vi "RFID Read Example.vi"() -> ()   [LabVIEW 2012, in "Phidget RFID.lvlib"]
uses:
  <instrlib>/Phidgets/Phidget RFID/Phidget RFID.lvlib
  <instrlib>/Phidgets/Phidget RFID/Public/RFIDStart.vi
  <instrlib>/Phidgets/Phidget RFID/Public/RFIDClose.vi
  <instrlib>/Phidgets/Phidget Common/Phidget Common.lvlib
panel:
  out "Protocol":i32(ring) items=["PROTOCOL_EM4100"=1, "PROTOCOL_ISO11785_FDX_B"=2, "PROTOCOL_PHIDGETS"=3]
  out "Tag String":string
  out "Tag Present":bool caption="Tag State"
  in  "stop":bool
  out "error out":errorcluster
  in  "error in (no error)":errorcluster
  in  "Device Info":T1={"Serial Number"=-1, "Channel"=0, "Port"=0}
  out "Attached?":bool
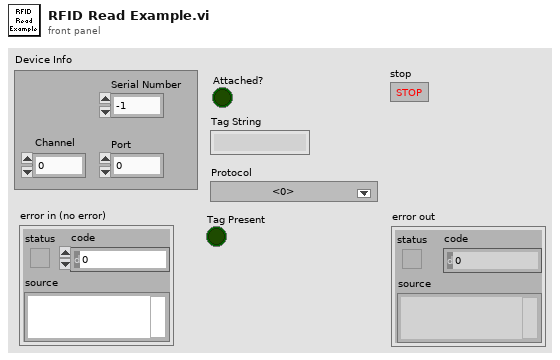
[diagram p1: front panel]
types:
  T1 = cluster{"Serial Number":i32, "Channel":i32, "Port":i32}
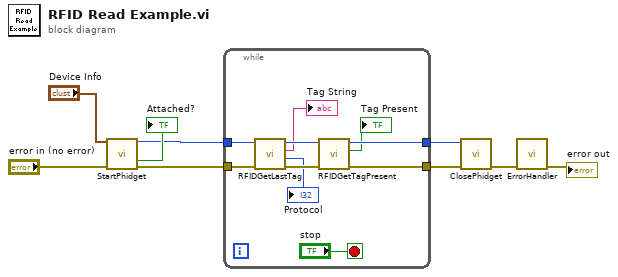
[diagram p0: block diagram]
diagram:
  n1 = call-poly <instrlib>:"StartPhidget.vi"("Device Info"="Device Info", "error in (no error)"="error in (no error)") -> ("Phidget ID"=w4:u64, "Attached?"=→"Attached?":bool, "error out"=w3:errorcluster)  [unwired: 10 in, 1 out]
  n2 = while {
    tunnel: w4 -> [w19]
    tunnel: w3 -> [w18]
    tunnel: [w15] -> w2
    tunnel: [w14] -> w1
    stop <- "stop" stop-if-true
    n3 = call <instrlib>:"RFIDGetLastTag.vi"("error in (no error)"=w18, "Device In"=w19) -> ("error out"=w16:errorcluster, "Protocol"=→"Protocol":i32, "Tag String"=→"Tag String":string, "Device Out"=w17:u64)  [unwired: 6 in]
    n4 = call <instrlib>:"RFIDGetTagPresent.vi"("error in (no error)"=w16, "Device In"=w17) -> ("error out"=w15:errorcluster, "Tag State"=→"Tag Present":bool, "Device Out"=w14:u64)  [unwired: 6 in]
  }
  n5 = call-poly <instrlib>:"ClosePhidget.vi"("error in"=w2, "Device In"=w1) -> ("error out"=w6:errorcluster)  [unwired: 9 in]
  n6 = call <instrlib>:"ErrorHandler.vi"("error in"=w6) -> ("error out"=→"error out":errorcluster)  [unwired: 9 in, 1 out]
